vi "CRYProject Editor PIC Event to MSG Proc.vi"(9 "nData":i32, 10 "sData":string="GVSMAIN_ACTION", 11 "sEventName":string="GVSMAIN_ACTION") -> ()   [LabVIEW 2013]
uses:
  CRYProject Editor Global.vi
  CRYWindow/SubVI/CRYMain Sub Window Global.vi
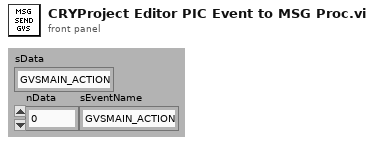
[diagram p1: front panel]
types:
  T1 = cluster{"EventName":string, "Arg1":string, "Numeric":u16, "Numeric 2":u16, "AddSteps ":refnum<vi>, "Arg1 2":string, "Arg1 3":string, "Boolean":bool}
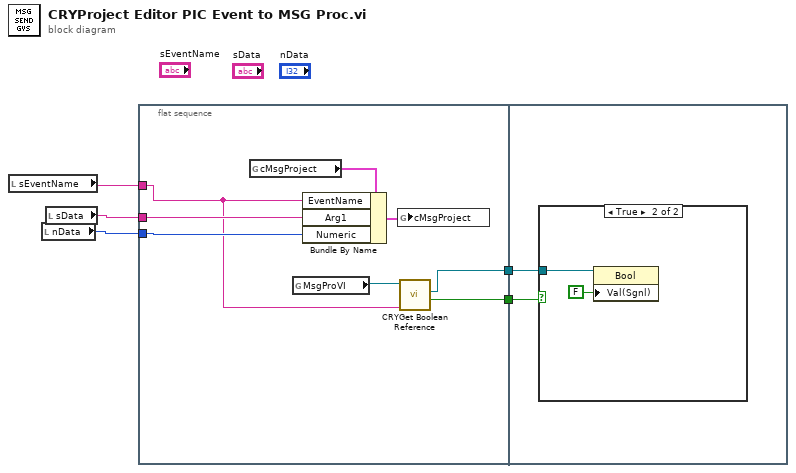
[diagram p0: block diagram]
diagram:
  n1 = local read "sEventName"() -> (w4:string)
  n2 = local read "nData"() -> (w3:i32)
  n3 = local read "sData"() -> (w5:string)
  n4 = flat-sequence {
    tunnel: w5 -> [w11]
    tunnel: w4 -> [w8]
    tunnel: w3 -> [w10]
    tunnel: [w7] -> w2
    tunnel: [w6] -> w1
    tunnel: w2 -> [w15]
    tunnel: w1 -> [w14]
    frame #0 {
      n5 = global read "CRYProject Editor Global.vi" "cMsgProject"() -> (w13:T1)
      n6 = global read "CRYMain Sub Window Global.vi" "MsgProVI"() -> (w9:refnum<vi>)
      n7 = Bundle By Name(cluster=w13, "EventName"=w8, "Arg1"=w11, "Numeric"=w10) -> (w12:T1)
      n8 = global write "CRYProject Editor Global.vi" "cMsgProject"(w12) -> ()
      n9 = call "CRYGet Boolean Reference.vi"("Label Name"=w8, "VI Refnum"=w9) -> ("Exist?"=w7:bool, "Boolean Ref"=w6:refnum<vi>)  [unwired: 7 in, 1 out]
    }
    frame #1 {
      n10 = case shown="True" w15 {
        tunnel: w14 -> [_ w17]
        frame False {
        }
        frame True {
          n11 = property class="Bool"(reference=w17, "Val(Sgnl)"=FALSE) -> ()  [unwired: 1 in, 2 out]
        }
      }
    }
  }
